vi "FPGA.vi"() -> ()   [LabVIEW 2017]
uses:
  <vilib>/rvi/Emulation/niFpgaGetClockAttributes.vi
  <vilib>/rvi/Emulation/niFpgaSctlEmulationGetInTimedLoop.vi
  <vilib>/rvi/Emulation/niFpgaEmulationReportErrorSimple.vi
  <vilib>/IEDriver/SPIandI2C/FPGA/Private/Initialize Port (I2C).vi
  <vilib>/IEDriver/SPIandI2C/FPGA/Private/IP Port (I2C).vi
  <vilib>/rvi/eio/common/nirviEmuTemplateMethod_errors.vi
  <vilib>/IEDriver/SPIandI2C/FPGA/Private/Configure Port (I2C).vi
  <vilib>/IEDriver/SPIandI2C/FPGA/Private/Read Port (I2C).vi
  <vilib>/IEDriver/SPIandI2C/FPGA/Private/Arm Port (I2C).vi
  <vilib>/IEDriver/SPIandI2C/FPGA/Private/Write Port (I2C).vi
  <vilib>/rvi/Emulation/niFpgaProcessEmulError.vi
  <vilib>/rvi/Emulation/niFpgaCriticalErrorInLSC.vi
  <vilib>/eio/EIONode/EIONode.xnode
  <vilib>/IEDriver/SPIandI2C/FPGA/Library/IP SPI&I2C.lvlib
panel:
  in  "I2C Protocol Action 0":T1(ring)=enum."Idle"
  in  "I2C Protocol Input Data 0":u8
  out "I2C Protocol Output Data 0":u8
  in  "I2C Protocol Configure 0":T2 {"Command (Write & Read)" items=["Write & Read", "Write", "Read"]}
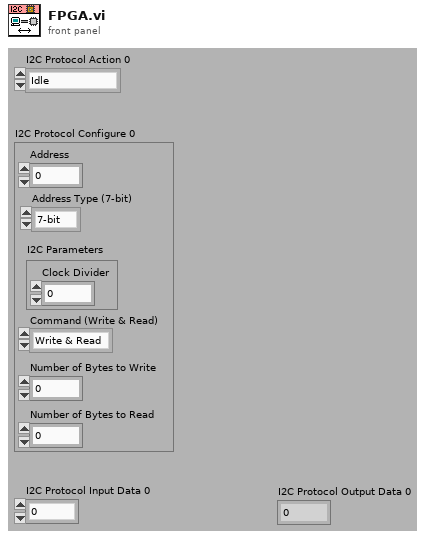
[diagram p1: front panel]
types:
  T1 = enum8{"Configure", "Write", "Arm", "Read", "Set Idle", "Idle"}
  T2 = cluster{"Address":u16, "Address Type (7-bit)":enum16{"7-bit", "10-bit"}, "I2C Parameters":cluster{"Clock Divider":u32}, "Command (Write & Read)":u8, "Number of Bytes to Write":u16, "Number of Bytes to Read":u16}
  T3 = typedef "IP SPI&I2C.lvlib/Private Data (I2C).ctl" = cluster{"Arm Trigger":refnum<k21>, "API to IP Data":refnum<k21>, "IP to API Data":refnum<k21>, "Configuration Register":refnum<k21>, "Configuration Lock":refnum<k21>}
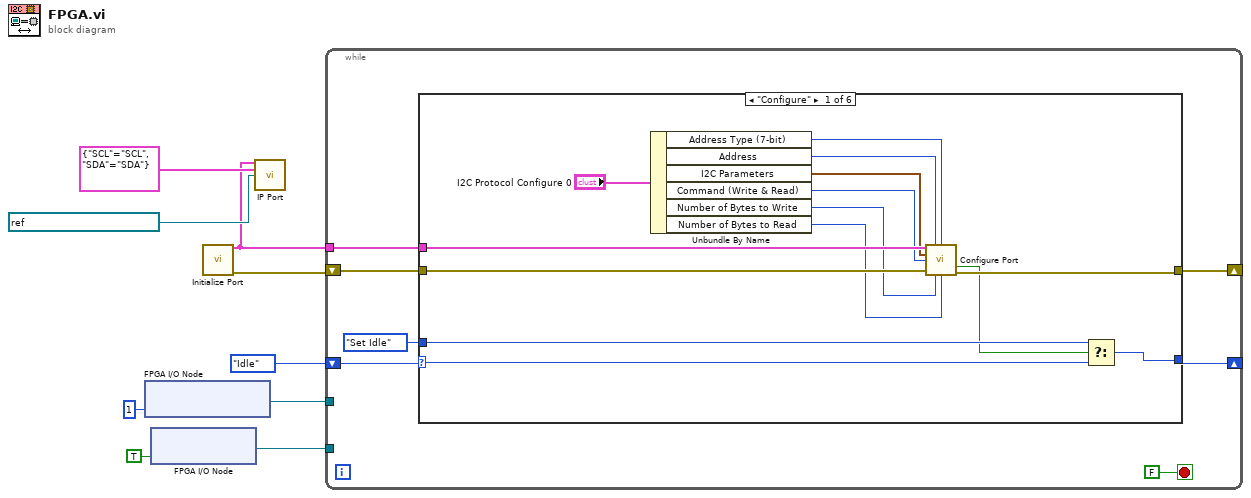
[diagram p0: block diagram]
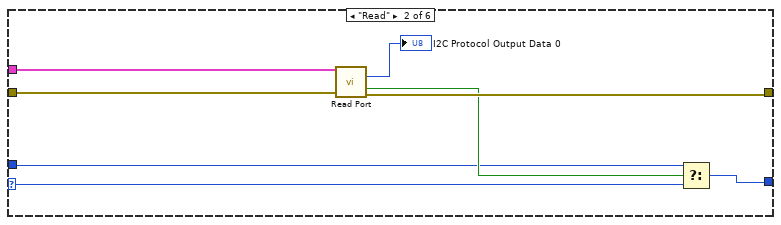
[diagram p2: hidden frame]
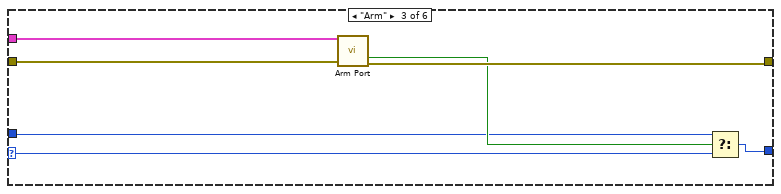
[diagram p3: hidden frame]
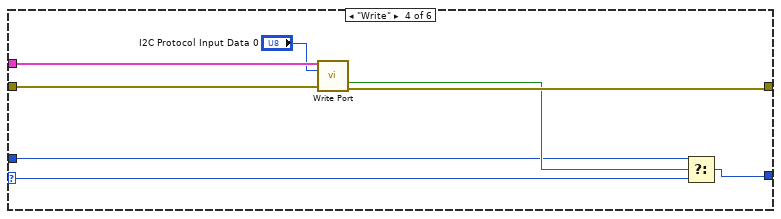
[diagram p4: hidden frame]
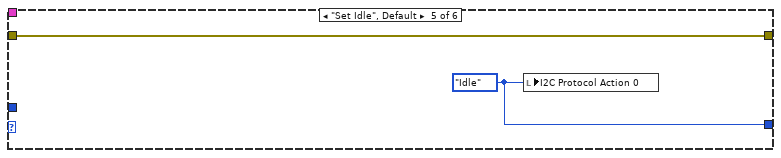
[diagram p5: hidden frame]
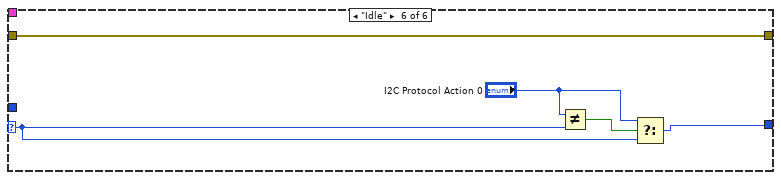
[diagram p6: hidden frame]
diagram:
  n1 = xnode "FPGA I/O Node"("USER FPGA LED"=u8 1) -> ("FPGA I/O Out"=w1:refnum<k21>)  [unwired: 1 in]
  n2 = xnode "FPGA I/O Node"("Mod7/DIO2"=TRUE ("Mod1/DIO1")) -> ("FPGA I/O Out"=w4:refnum<k21>)  [unwired: 1 in]
  n3 = call-poly <vilib>:"Initialize Port.vi"() -> ("Private Data Out"=w7:T3, "error out"=w6:errorcluster)  [unwired: 14 in]
  n4 = call-poly <vilib>:"IP Port.vi"("Private Data In"=w7, "I2C FPGA IO"=cluster{"SCL":refnum<k21>, "SDA":refnum<k21>} {"SCL"="SCL", "SDA"="SDA"}, "FPGA Clock"=refnum<k21> "40 MHz Onboard Clock") -> ()  [unwired: 13 in]
  n5 = while {
    shift-right: [w13] -> _
    shift-left: w6 -> [w15]
    tunnel: w7 -> [w16]
    shift-right: [w11] -> _
    shift-left: T1."Idle" ("Action") -> [w12]
    tunnel: w4 -> [_]
    tunnel: w1 -> [_]
    stop <- FALSE stop-if-true
    n6 = case shown="\"Configure\"" w12 {
      selector: w12 -> [w21 w32 w40 w47 _ w57]
      tunnel: w16 -> [w30 w38 w45 w53 _ _]
      tunnel: w15 -> [w29 w37 w44 w52 w55 w60]
      tunnel: [w28 w36 w43 w51 w55 w60] -> w13
      tunnel: [w22 w34 w42 w48 w54 w56] -> w11
      tunnel: T1."Set Idle" ("Action") -> [w20 w31 w39 w46 _ _]
      frame "Configure" {
        n7 = Unbundle By Name("I2C Protocol Configure 0") -> ("Address Type (7-bit)"=w26:enum16{"7-bit", "10-bit"}, "Address"=w17:u16, "I2C Parameters"=w25:cluster{"Clock Divider":u32}, "Command (Write & Read)"=w18:u8, "Number of Bytes to Write"=w24:u16, "Number of Bytes to Read"=w23:u16)
        n8 = call-poly <vilib>:"Configure Port.vi"("Private Data In"=w30, "Address"=w17, "Address Type (7-bit)"=w26, "I2C Parameters"=w25, "Command (Write & Read)"=w18, "error in"=w29, "Number of Bytes to Write"=w24, "Number of Bytes to Read"=w23) -> ("Done"=w19:bool, "error out"=w28:errorcluster)  [unwired: 5 in, 1 out]
        n9 = Select(t=w20, s=w19, f=w21) -> (s? t:f=w22:T1)
      }
      frame "Read" {
        n10 = call-poly <vilib>:"Read Port.vi"("Private Data In"=w38, "error in"=w37) -> ("Data Out"=→"I2C Protocol Output Data 0":u8, "Output Valid"=w33:bool, "error out"=w36:errorcluster)  [unwired: 10 in, 1 out]
        n11 = Select(t=w31, s=w33, f=w32) -> (s? t:f=w34:T1)
      }
      frame "Arm" {
        n12 = call-poly <vilib>:"Arm Port.vi"("Private Data In"=w45, "error in"=w44) -> ("Done"=w41:bool, "error out"=w43:errorcluster)  [unwired: 11 in, 1 out]
        n13 = Select(t=w39, s=w41, f=w40) -> (s? t:f=w42:T1)
      }
      frame "Write" {
        n14 = call-poly <vilib>:"Write Port.vi"("Private Data In"=w53, "Data In"="I2C Protocol Input Data 0", "error in"=w52) -> ("Done"=w49:bool, "error out"=w51:errorcluster)  [unwired: 10 in, 1 out]
        n15 = Select(t=w46, s=w49, f=w47) -> (s? t:f=w48:T1)
      }
      frame "Set Idle", Default {
        w54 = T1."Idle" ("Action")
        n16 = local write "I2C Protocol Action 0"(w54) -> ()
      }
      frame "Idle" {
        n17 = Not Equal?(x="I2C Protocol Action 0", y=w57) -> (x != y?=w59:bool)
        n18 = Select(t="I2C Protocol Action 0", s=w59, f=w57) -> (s? t:f=w56:T1)
      }
    }
  }
